vi "Servo MSMT ET Set RF Power.vi"(8 "error in (no error)":errorcluster, 10 "Step In":refnum<k7>, 11 "Servo MSMT in":refnum<class "Servo MSMT.lvclass">) -> (0 "error out":errorcluster, 2 "Step Out":refnum<k7>, 3 "Servo MSMT out":refnum<class "Servo MSMT.lvclass">)   [LabVIEW 2018, in "Servo MSMT.lvlib" / "Servo MSMT.lvclass"]
uses:
  Servo MSMT.lvclass
  Plugins/String Database.lvlibp/String Database.lvclass
  Plugins/TestStand API Tools (TSAT).lvlibp/Step Actions/TSAT Step Actions.lvlib
  Plugins/Test Group Manager.lvlibp/Test Group Manager.lvclass
  Plugins/Test Group Manager.lvlibp/Includes/Test Group/Test Group.lvclass
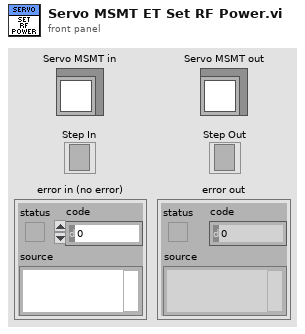
[diagram p1: front panel]
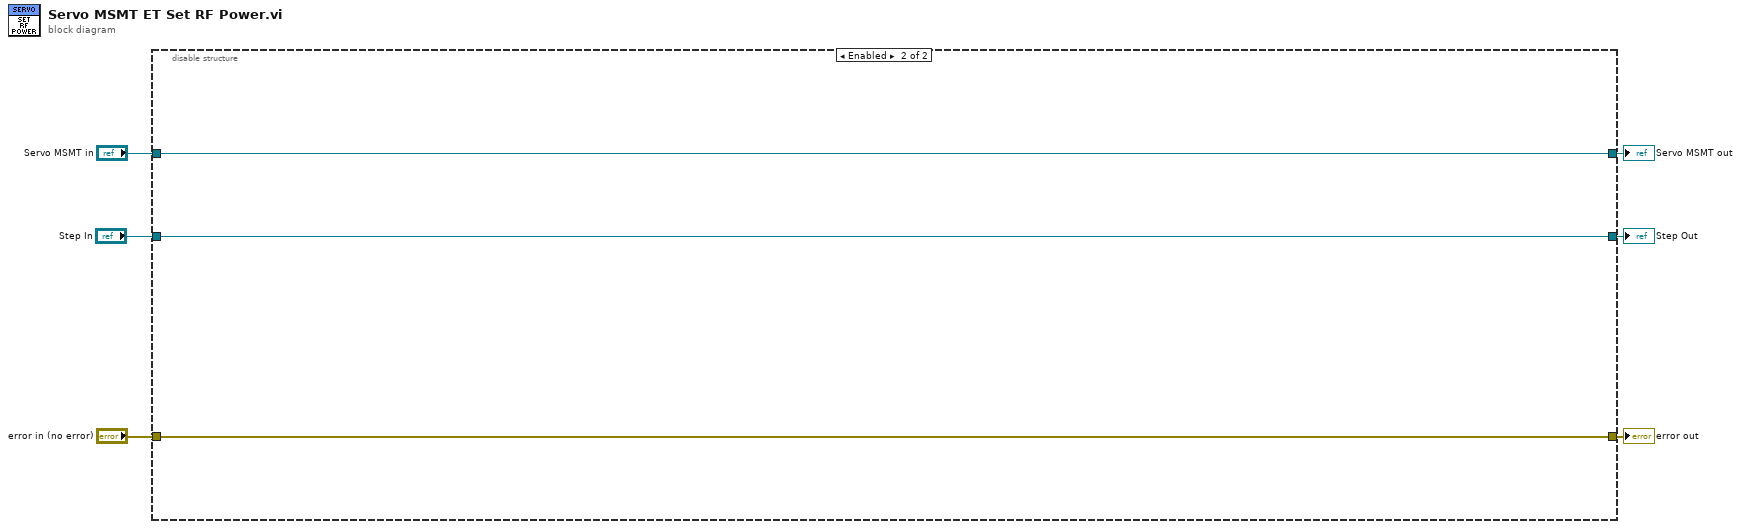
[diagram p0: block diagram]
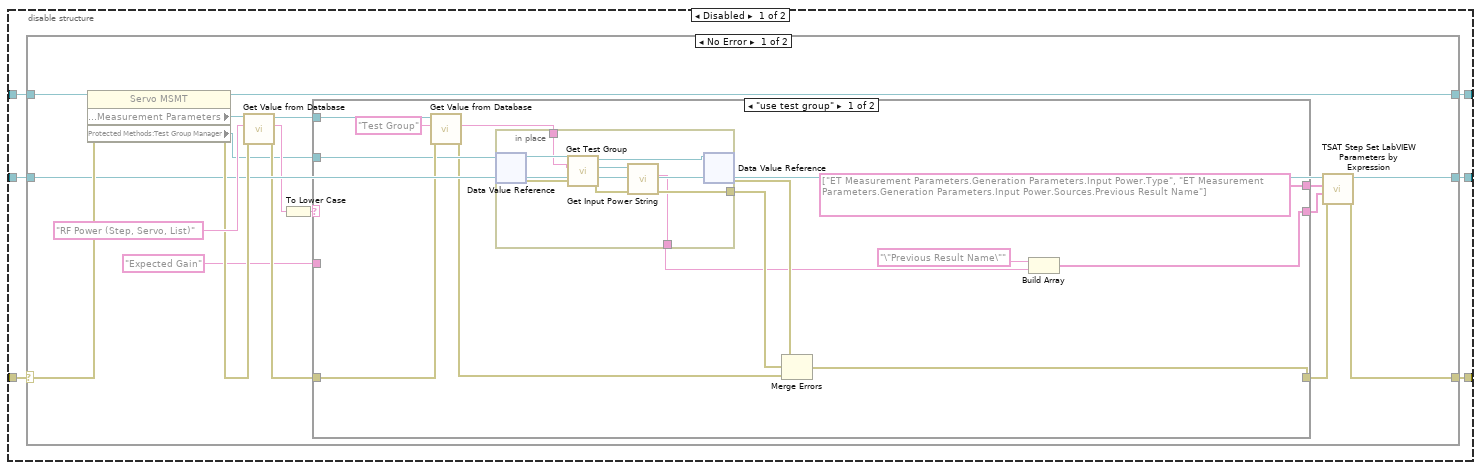
[diagram p2: hidden frame]
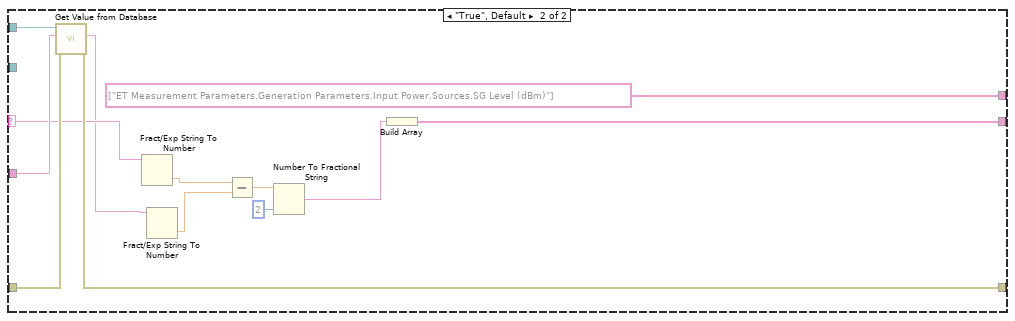
[diagram p3: hidden frame]
diagram:
  n1 = disable-structure shown="Enabled" {
    disable-tunnel: "error in (no error)" -> [w12 w68]
    disable-tunnel: [w11 w68] -> w5
    disable-tunnel: "Servo MSMT in" -> [w10 w70]
    disable-tunnel: [w9 w70] -> w3
    disable-tunnel: "Step In" -> [w8 w69]
    disable-tunnel: [w7 w69] -> w1
    frame Disabled {
      n2 = case shown="No Error" w12 {
        selector: w12 -> [w30 w67]
        tunnel: [w22 w67] -> w11
        tunnel: [w28 w66] -> w9
        tunnel: w10 -> [w29 w66]
        tunnel: w8 -> [w24 w65]
        tunnel: [w23 w65] -> w7
        frame No Error {
          n3 = property class="Servo MSMT"(reference=w29, error in=w30) -> (reference out=w28:refnum<class "Servo MSMT.lvclass">, error out=w25:errorcluster, "Protected Methods:Measurement Parameters"=w27:refnum<class "String Database.lvclass">, "Protected Methods:Test Group Manager"=w13:refnum<data-value>)
          n4 = call "Get Value from Database.vi"("error in (no error)"=w25, "Entry Name"="RF Power (Step, Servo, List)", "Message in"=w27) -> ("error out"=w18:errorcluster, "Entry Value"=w15:string, "Message out"=w19:refnum<class "String Database.lvclass">)  [unwired: 5 in, 1 out]
          n5 = To Lower Case(string=w15) -> (all lower case string=w14:string)
          n6 = case shown="\"use test group\"" w14 {
            selector: w14 -> [_ w58]
            tunnel: [string[] ["ET Measurement Parameters.Generation Parameters.Input Power.Type", "ET Measurement Parameters.Generation Parameters.Input Power.Sources.Previous Result Name"] ("Parameters to Set") string[] ["ET Measurement Parameters.Generation Parameters.Input Power.Sources.SG Level (dBm)"] ("Parameters to Set")] -> w21
            tunnel: [w31 w63] -> w20
            tunnel: w19 -> [w43 w62]
            tunnel: w18 -> [w42 w61]
            tunnel: [w37 w60] -> w17
            tunnel: "Expected Gain" ("Entry Name") -> [_ w59]
            tunnel: w13 -> [w40 _]
            frame "use test group" {
              n7 = call "Get Value from Database.vi"("error in (no error)"=w42, "Entry Name"="Test Group", "Message in"=w43) -> ("error out"=w38:errorcluster, "Entry Value"=w39:string)  [unwired: 5 in, 2 out]
              n8 = in-place {
                in-place-border: w39 -> [w49]
                in-place-border: [w45] -> w35
                in-place-border: [w44] -> w32
                n9 = in-place-dvr #1(w40) -> (w51:refnum<class "Test Group Manager.lvclass">, w50:errorcluster)
                n10 = call "Get Test Group.vi"("error in (no error)"=w50, "Test Group Name"=w49, "Test Group Manager in"=w51) -> ("error out"=w48:errorcluster, "Test Group In"=w47:refnum<data-value>, "Test Group Manager out"=w46:refnum<class "Test Group Manager.lvclass">)  [unwired: 6 in]
                n11 = call "Get Input Power String.vi"("error in (no error)"=w48, "Test Group In"=w47) -> ("error out"=w45:errorcluster, "Input Power"=w44:string)  [unwired: 7 in, 1 out]
                n12 = in-place-dvr #1(w46) -> (w36:errorcluster)  [unwired: 1 out]
              }
              n13 = Merge Errors(w36, w35, w38) -> (w37:errorcluster)
              n14 = Build Array("\"Previous Result Name\"", w32) -> (w31:string[])
            }
            frame "True", Default {
              n15 = call "Get Value from Database.vi"("error in (no error)"=w61, "Entry Name"=w59, "Message in"=w62) -> ("error out"=w60:errorcluster, "Entry Value"=w57:string)  [unwired: 5 in, 2 out]
              n16 = Fract/Exp String To Number(string=w58) -> (number=w56:dbl)  [unwired: 3 in, 1 out]
              n17 = Fract/Exp String To Number(string=w57) -> (number=w55:dbl)  [unwired: 3 in, 1 out]
              n18 = Subtract(x=w56, y=w55) -> (x-y=w54:dbl)
              n19 = Number To Fractional String(number=w54, precision (6)=i16 2) -> (F-format string=w52:string)  [unwired: 2 in]
              n20 = Build Array(w52) -> (w63:string[])
            }
          }
          n21 = call "TSAT Step Set LabVIEW Parameters by Expression.vi"("Error In"=w17, "Value Expressions"=w20, "Parameters to Set"=w21, "Step In"=w24) -> ("Error Out"=w22:errorcluster, "Step Out"=w23:refnum<k7>)  [unwired: 6 in]
        }
        frame Error {
        }
      }
    }
    frame Enabled {
    }
  }
  "error out" <- w5
  "Servo MSMT out" <- w3
  "Step Out" <- w1
